vi "zipped-dataset.vi"() -> ()   [LabVIEW 2018]
uses:
  <vilib>/addons/h5labview2/file/H5Fmode.ctl
  HDF5/lib_path_mod_20200519.vi
  <vilib>/addons/h5labview2/base/H5Equery.vi
  <vilib>/addons/h5labview2/dataset/H5Dwrite.llb/H5Dwrite.xnode
  <vilib>/addons/h5labview2/file/H5F.lvlib
  <vilib>/addons/h5labview2/space/H5S.lvlib
  <vilib>/addons/h5labview2/type/H5T.lvlib
  <vilib>/addons/h5labview2/props/H5P.lvlib
  <vilib>/addons/h5labview2/dataset/H5D.lvlib
panel:
  out "Count":i32
  in  "Numeric":dbl
  out "error out":errorcluster
  in  "data":dbl[](array[numeric])
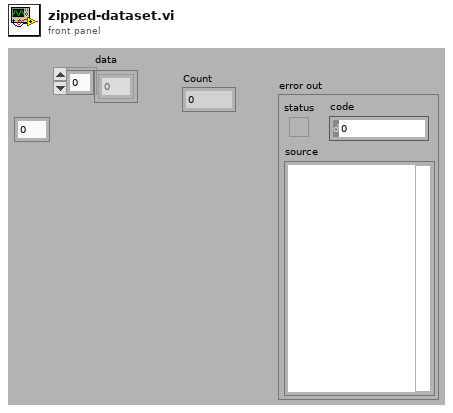
[diagram p1: front panel]
types:
  T1 = typedef "H5F.lvlib/H5Fmode.ctl" = enum16{"read-only", "read-write", "overwrite", "create new", "open or create"}
  T2 = typedef "hid_t.ctl" = i32
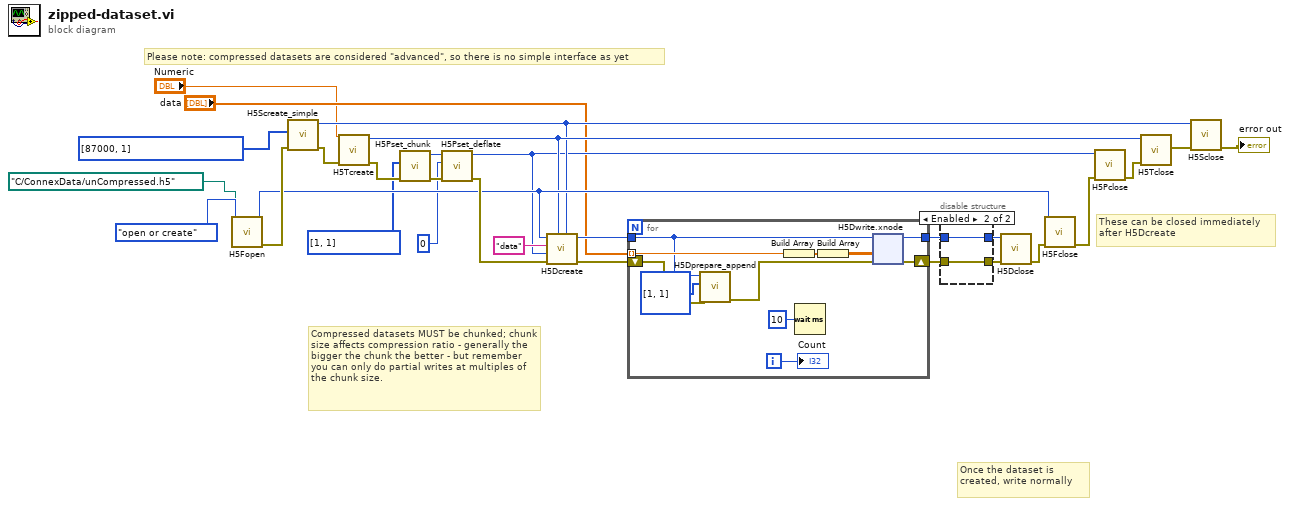
[diagram p0: block diagram]
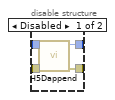
[diagram p2: hidden frame]
diagram:
  # "Please note: compressed datasets are considered \"advanced\", so there is no simple interface as yet"
  # "Once the dataset is created, write normally"
  # "Compressed datasets MUST be chunked; chunk size affects compression ratio - generally the bigger the chunk the better - but remember you can only do partial writes at multiples of the chunk size."
  # "These can be closed immediately after H5Dcreate"
  n1 = call <vilib>:"H5Fopen.vi"("mode (read-only)"=H5Fmode."open or create" ("mode"), "path"=path "C:/ConnexData/unCompressed.h5" ("name or relative path")) -> ("error out"=w24:errorcluster, "ref out"=w23:T2)  [unwired: 8 in]
  n2 = call <vilib>:"H5Screate_simple.vi"("error in (no error)"=w24, "maxdims"=u64[] [87000, 1]) -> ("error out"=w27:errorcluster, "space out"=w18:T2)  [unwired: 7 in, 1 out]
  n3 = call <vilib>:"H5Tcreate.vi"("error in (no error)"=w27, "type variant"="Numeric") -> ("error out"=w10:errorcluster, "type out"=w19:i32)  [unwired: 7 in, 1 out]
  n4 = call <vilib>:"H5Pset_chunk.vi"("error in (no error)"=w10, "chunk size"=u32[] [1, 1]) -> ("error out"=w9:errorcluster, "prop out"=w8:T2)  [unwired: 8 in]
  n5 = call <vilib>:"H5Pset_deflate.vi"("error in (no error)"=w9, "level"=u8 0, "prop in"=w8) -> ("error out"=w26:errorcluster, "prop out"=w15:T2)  [unwired: 7 in]
  n6 = call <vilib>:"H5Dcreate.vi"("space id"=w18, "type id"=w19, "error in (no error)"=w26, "props id"=w15, "name"="data", "loc in"=w23) -> ("error out"=w22:errorcluster, "dset out"=w21:T2)  [unwired: 2 in]
  n7 = for {
    tunnel: w21 -> [w33]
    tunnel: [w39] -> w3
    tunnel: "data" -> [w38] mode=indexing
    shift-right: [w40] -> w2
    shift-left: w22 -> [w32]
    i -> [w34]
    n8 = call <vilib>:"H5Dprepare_append.vi"("error in (no error)"=w32, "append dims"=u64[] [1, 1], "dset in"=w33) -> ("error out"=w31:errorcluster)  [unwired: 5 in, 3 out]
    n9 = Build Array(w38) -> (w36:dbl[])
    n10 = Wait (ms)(milliseconds to wait=u32 10) -> ()  [unwired: 1 out]
    n11 = Build Array(w36) -> (w35:dbl[][])
    n12 = xnode "H5Dwrite.xnode"("error in (no error)"=w31, "data"=w35, "ref in"=w33) -> ("error out"=w40:errorcluster, "ref out"=w39:i32)  [unwired: 4 in, 1 out]
    "Count" <- w34
  }
  n13 = disable-structure shown="Enabled" {
    disable-tunnel: [w63 w65] -> w20
    disable-tunnel: w3 -> [w62 w65]
    disable-tunnel: w2 -> [w61 w64]
    disable-tunnel: [w60 w64] -> w1
    frame Disabled {
      n14 = call <vilib>:"H5Dappend.vi"("error in (no error)"=w61, "ref in"=w62) -> ("error out"=w60:errorcluster, "ref out"=w63:T2)  [unwired: 6 in, 2 out]
    }
    frame Enabled {
    }
  }
  n15 = call <vilib>:"H5Dclose.vi"("error in (no error)"=w1, "dset in"=w20) -> ("error out"=w14:errorcluster)  [unwired: 9 in]
  n16 = call <vilib>:"H5Fclose.vi"("error in (no error)"=w14, "ref"=w23) -> ("error out"=w13:errorcluster)  [unwired: 9 in]
  n17 = call <vilib>:"H5Pclose.vi"("error in (no error)"=w13, "props in"=w15) -> ("error out"=w16:errorcluster)  [unwired: 9 in]
  n18 = call <vilib>:"H5Tclose.vi"("error in (no error)"=w16, "type in"=w19) -> ("error out"=w17:errorcluster)  [unwired: 9 in]
  n19 = call <vilib>:"H5Sclose.vi"("error in (no error)"=w17, "space in"=w18) -> ("error out"=→"error out":errorcluster)  [unwired: 9 in]
